vi "3.1.14-Generate Act Angle Array.vi"(1 "Enum":T1(ring)=enum."Desired Change in Heading") -> (0 "Array":dbl[](array[numeric]))   [LabVIEW 2010]
uses:
  3.0-Global.vi
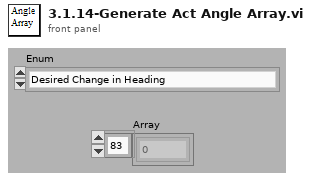
[diagram p1: front panel]
types:
  T1 = enum16{"Steering Setpoints", "Desired Change in Heading"}
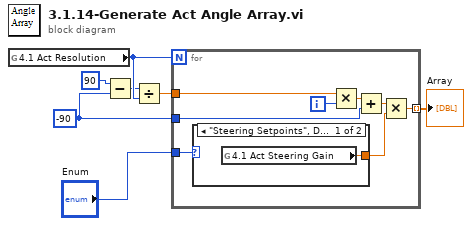
[diagram p0: block diagram]
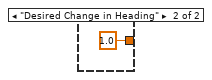
[diagram p2: hidden frame]
diagram:
  w5 = -90 ("y")
  n1 = global read "3.0-Global.vi" "4.1 Act Resolution"() -> (w7:u32)
  n2 = Subtract(x=90 ("y"), y=w5) -> (x-y=w3:i32)
  n3 = Divide(x=w3, y=w7) -> (x/y=w4:dbl)
  n4 = for {
    N: w7 -> [_]
    tunnel: [w10] -> w6 mode=indexing
    tunnel: w4 -> [w14]
    tunnel: w5 -> [w12]
    tunnel: "Enum" -> [w8]
    i -> [w11]
    n5 = case shown="\"Steering Setpoints\", Default" w8 {
      tunnel: [w16 1.0 ("4.1 Act Steering Gain")] -> w9
      frame "Steering Setpoints", Default {
        n6 = global read "3.0-Global.vi" "4.1 Act Steering Gain"() -> (w16:dbl)
      }
      frame "Desired Change in Heading" {
      }
    }
    n7 = Multiply(x=w14, y=w11) -> (x*y=w15:dbl)
    n8 = Add(x=w15, y=w12) -> (x+y=w13:dbl)
    n9 = Multiply(x=w13, y=w9) -> (x*y=w10:dbl)
  }
  "Array" <- w6
